vi "Calculate Radius (ball pick up).vi"(8 "Ball Y":dbl, 9 "Ball X":dbl, 10 "Min Detect Distance":dbl) -> (1 "Radius":dbl, 2 "X of intersection":dbl)   [LabVIEW 2015]
uses:
  <vilib>/express/express arith-compare/Formula/XNode/ExpressFormulaBlockNode.xnode
panel:
  in  "math tolerance":dbl=0.001
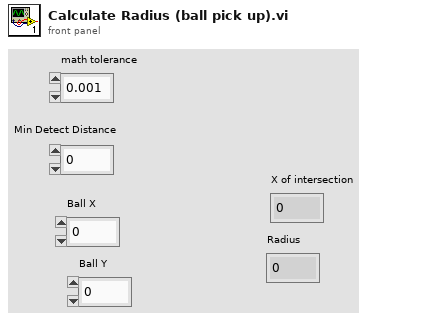
[diagram p1: front panel]
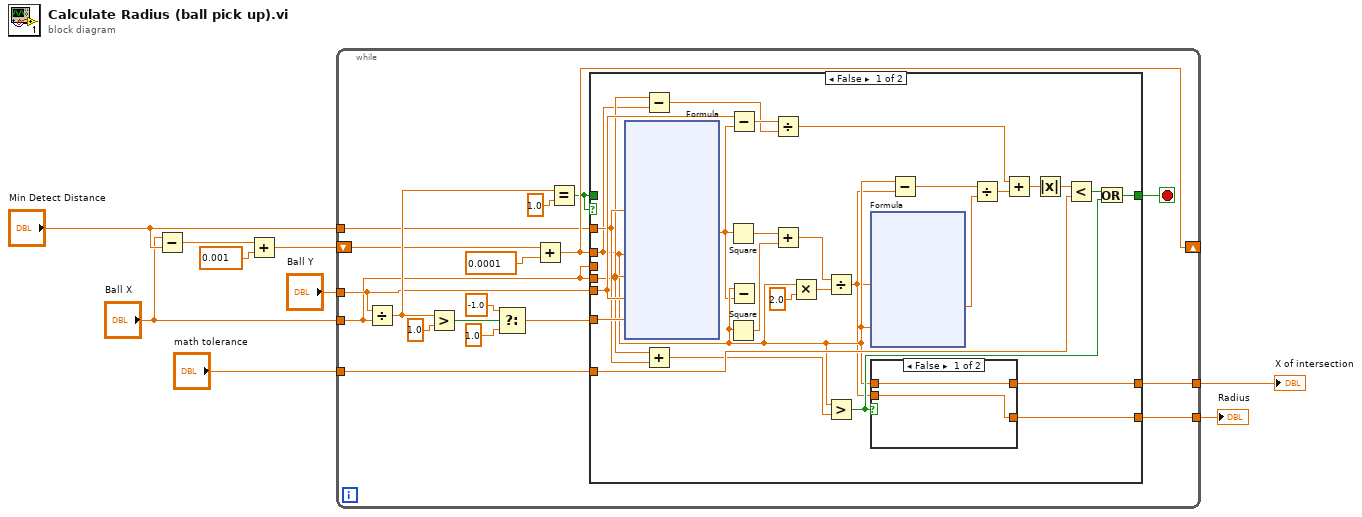
[diagram p0: block diagram]
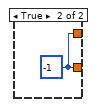
[diagram p2: hidden frame]
diagram:
  n1 = Subtract(x="Ball X", y="Min Detect Distance") -> (x-y=w9:dbl)
  n2 = Add(x=w9, y=0.001) -> (x+y=w2:dbl)
  n3 = while {
    shift-right: [w21] -> _
    shift-left: w2 -> [w12]
    tunnel: "Ball Y" -> [w22]
    tunnel: "math tolerance" -> [w16]
    tunnel: [w24] -> w6
    tunnel: [w23] -> w5
    tunnel: "Min Detect Distance" -> [w10]
    tunnel: "Ball X" -> [w11]
    stop <- w15 stop-if-true
    n4 = Divide(x=w22, y=w11) -> (x/y=w26:dbl)
    n5 = Greater?(x=w26, y=1.0) -> (0:w20:bool)
    n6 = Select(t=-1.0, s=w20, f=1.0) -> (s? t:f=w17:dbl)
    n7 = Add(x=w12, y=0.0001) -> (x+y=w21:dbl)
    n8 = Equal?(x=w26, y=1.0) -> (x = y?=w14:bool)
    n9 = case shown="False" w14 {
      tunnel: [w39 w84] -> w24
      tunnel: w11 -> [_ w84]
      tunnel: [w38 w84] -> w23
      tunnel: w10 -> [w34 _]
      tunnel: w11 -> [w32 _]
      tunnel: w22 -> [w48 _]
      tunnel: w21 -> [w30 _]
      tunnel: w17 -> [w49 _]
      tunnel: w16 -> [w40 _]
      tunnel: [w35 w85] -> w15
      tunnel: w14 -> [_ w85]
      frame False {
        n10 = xnode "Formula"("D"=w34, "X"=w30, "A"=w32, "B"=w48, "C"=w49) -> ("Result"=w29:dbl)  [unwired: 1 in, 1 out]
        n11 = Subtract(x=w32, y=w30) -> (x-y=w31:dbl)
        n12 = Add(x=w32, y=w34) -> (x+y=w33:dbl)
        n13 = Square(x=w29) -> (x^2=w54:dbl)
        n14 = Square(x=w30) -> (x^2=w53:dbl)
        n15 = Subtract(x=w48, y=w29) -> (x-y=w47:dbl)
        n16 = Subtract(x=w30, y=w29) -> ()  [unwired: 1 out]
        n17 = Divide(x=w47, y=w31) -> (x/y=w46:dbl)
        n18 = Add(x=w54, y=w53) -> (x+y=w52:dbl)
        n19 = Multiply(x=w30, y=2.0) -> (x*y=w50:dbl)
        n20 = Divide(x=w52, y=w50) -> (x/y=w28:dbl)
        n21 = Greater?(x=w30, y=w33) -> (0:w36:bool)
        n22 = xnode "Formula"("R"=w28, "X"=w30) -> ("Result"=w44:dbl)  [unwired: 1 in, 1 out]
        n23 = case shown="False" w36 {
          tunnel: [w56 w57] -> w39
          tunnel: w30 -> [w56 _]
          tunnel: [w55 w57] -> w38
          tunnel: w28 -> [w55 _]
          frame False {
          }
          frame True {
            w57 = -1
          }
        }
        n24 = Subtract(x=w30, y=w28) -> (x-y=w45:dbl)
        n25 = Divide(x=w45, y=w44) -> (x/y=w43:dbl)
        n26 = Add(x=w46, y=w43) -> (x+y=w42:dbl)
        n27 = Absolute Value(x=w42) -> (abs(x)=w41:dbl)
        n28 = Less?(x=w41, y=w40) -> (x < y?=w37:bool)
        n29 = Or(x=w37, y=w36) -> (x .or. y?=w35:bool)
      }
      frame True {
      }
    }
  }
  "Radius" <- w5
  "X of intersection" <- w6
